vi "Progress Bar Front Panel.vi"(7 "Enable Cancel?":bool, 9 "Main Title":string, 10 "Progress Bar Dialog":refnum<class "Progress Bar Dialog.lvclass">, 11 "Total":i32) -> ()   [LabVIEW 2020, in "Progress Bar Dialog.lvclass"]
uses:
  <vilib>/ProgressBar/Progress Bar Dialog.lvclass
  <vilib>/ProgressBar/Progress Bar Dialog.lvclass/Progress Bar Dialog.ctl
panel:
  in  "Cancelling":string="Cancelling..."
  in  "Progress Format String":string="%d of %s"
  out "Main Heading":string="Working..."
  in  "Cancel":bool
  out "Status Heading":string="0 of 0"
  out "Progress Bar":dbl(slide) scale=0.0..1.0
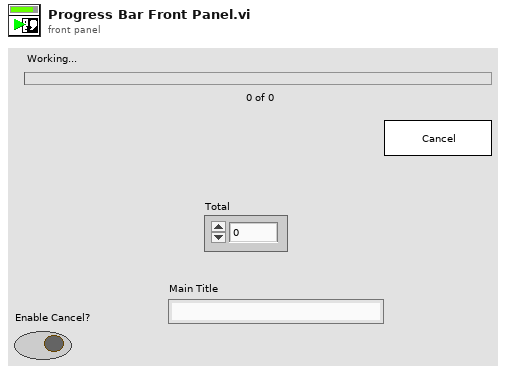
[diagram p1: front panel]
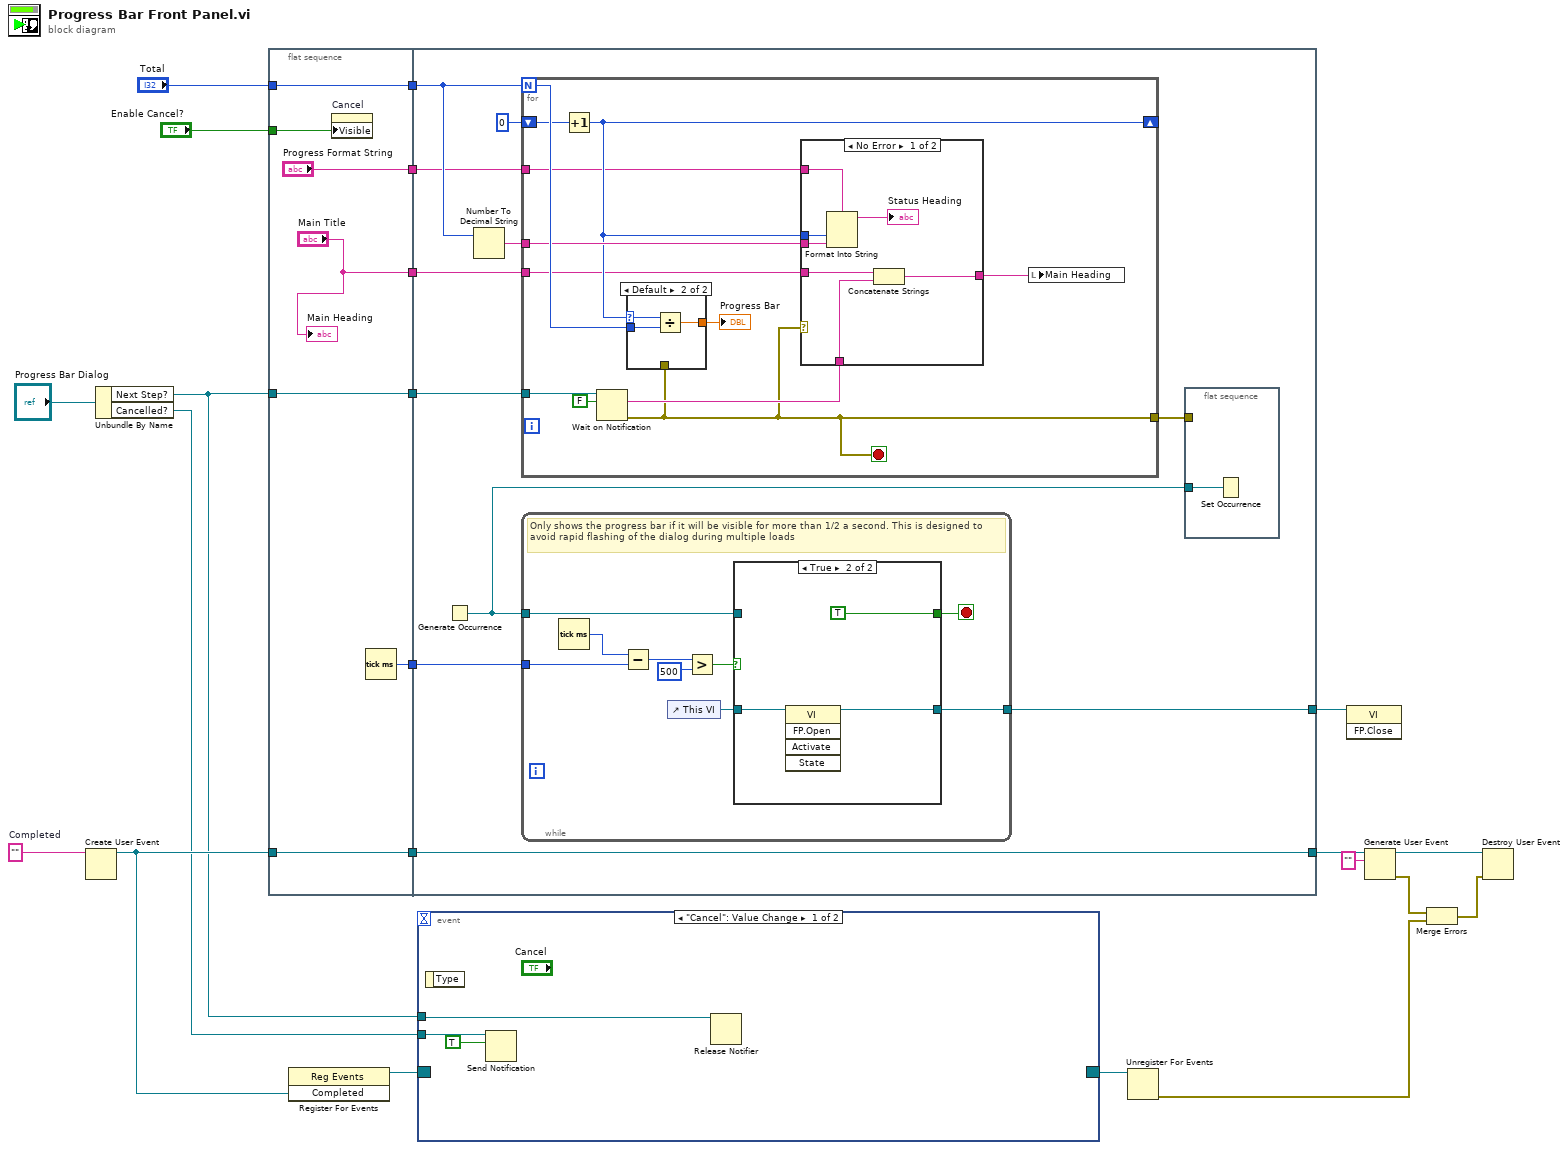
[diagram p0: block diagram]
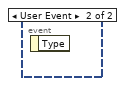
[diagram p2: hidden frame]
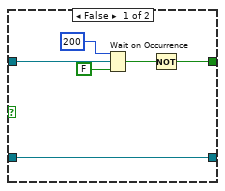
[diagram p3: hidden frame]
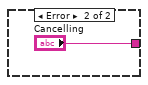
[diagram p4: hidden frame]
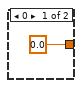
[diagram p5: hidden frame]
diagram:
  w13 = ""  # Completed
  n1 = Create User Event(user event datatype=w13) -> (user event=w15:refnum<user-event>)  [unwired: 1 in, 1 out]
  n2 = Unbundle By Name("Progress Bar Dialog") -> ("Next Step?"=w8:refnum<notifier>, "Cancelled?"=w7:refnum<notifier>)
  n3 = flat-sequence {
    tunnel: [w29] -> w22
    tunnel: [w28] -> w21
    tunnel: "Total" -> [w28]
    tunnel: "Enable Cancel?" -> [w27]
    tunnel: [w26] -> w18
    tunnel: w8 -> [w26]
    tunnel: [w25] -> w16
    tunnel: w15 -> [w25]
    tunnel: ["Progress Format String"] -> w5
    tunnel: ["Main Title"] -> w2
    tunnel: w22 -> [w37]
    tunnel: w21 -> [w36]
    tunnel: w18 -> [w35]
    tunnel: [w34] -> w14
    tunnel: w16 -> [w34]
    tunnel: [w32] -> w6
    tunnel: w5 -> [w31]
    tunnel: w2 -> [w30]
    frame #0 {
      n4 = property on="Cancel" class="Bool"("Visible"=w27) -> ()  [unwired: 2 in, 2 out]
      n5 = Tick Count (ms)() -> (millisecond timer value=w29:u32)
      "Main Heading" <- "Main Title"
    }
    frame #1 {
      n6 = Generate Occurrence() -> (w38:refnum<k4>)
      n7 = Number To Decimal String(number=w36) -> (decimal integer string=w39:string)  [unwired: 1 in]
      n8 = for {
        N: w36 -> [w71]
        shift-right: [w64] -> _
        shift-left: 0 -> [w66]
        tunnel: w35 -> [w69]
        tunnel: w39 -> [w68]
        tunnel: [w60] -> w33
        tunnel: w31 -> [w63]
        tunnel: w30 -> [w62]
        stop <- w60 stop-if-true
        n9 = Increment(x=w66) -> (x+1=w64:i32)
        n10 = Wait on Notification(notifier=w69, ignore previous (F)=FALSE) -> (notification=w65:string, error out=w60:errorcluster)  [unwired: 2 in, 2 out]
        n11 = case shown="Default" w64 {
          selector: w64 -> [_ w83]
          tunnel: w71 -> [_ w82]
          tunnel: [0.0 w81] -> w70
          tunnel: w60 -> [_ _]
          frame 0 {
          }
          frame Default {
            n12 = Divide(x=w83, y=w82) -> (x/y=w81:dbl)
          }
        }
        "Progress Bar" <- w70
        n13 = case shown="No Error" w60 {
          tunnel: w68 -> [w78 _]
          tunnel: w65 -> [w74 _]
          tunnel: w64 -> [w77 _]
          tunnel: w63 -> [w76 _]
          tunnel: w62 -> [w75 _]
          tunnel: [w73 "Cancelling"] -> w61
          frame No Error {
            n14 = Format Into String(format string=w76, w77, w78) -> (resulting string=→"Status Heading":string)  [unwired: 2 in, 1 out]
            n15 = Concatenate Strings(w75, w74) -> (w73:string)
          }
          frame Error {
          }
        }
        n16 = local write "Main Heading"(w61) -> ()
      }
      n17 = while {
        tunnel: w38 -> [w42]
        tunnel: w37 -> [w47]
        tunnel: [w45] -> w32
        stop <- w43 stop-if-true
        # "Only shows the progress bar if it will be visible for more than 1/2 a second. This is designed to avoid rapid flashing of the dialog during multiple loads"
        n18 = Tick Count (ms)() -> (millisecond timer value=w48:u32)
        n19 = Subtract(x=w48, y=w47) -> (x-y=w49:u32)
        n20 = control-ref of="This VI"() -> (w46:refnum<vi>)
        n21 = Greater?(x=w49, y=u32 500) -> (0:w44:bool)
        n22 = case shown="True" w44 {
          tunnel: w46 -> [w56 w59]
          tunnel: [w56 w58] -> w45
          tunnel: [w51 TRUE] -> w43
          tunnel: w42 -> [w53 _]
          frame False {
            n23 = Wait on Occurrence(1:FALSE ("ignore previous (T)"), 2:w53, 3:200 ("ms timeout (-1)")) -> (0:w52:bool)
            n24 = Not(x=w52) -> (.not. x?=w51:bool)
          }
          frame True {
            n25 = invoke class="VI" method="FP.Open"(reference=w59) -> (reference out=w58:refnum<vi>)  [unwired: 4 in, 4 out]
          }
        }
      }
      n26 = flat-sequence {
        tunnel: w38 -> [w41]
        tunnel: w33 -> [_]
        frame #0 {
          n27 = Set Occurrence(w41) -> ()
        }
      }
    }
  }
  n28 = register-events(w15) -> (reference out=w17:refnum<event-registration>)  [unwired: 2 in, 1 out]
  n29 = event shown="[0] \"Cancel\": Value Change" {
    selector: w17 -> [_ _]
    dyn-events: [_ _] -> w4
    timeout: _ -> [_ _]
    tunnel: w8 -> [w86 _]
    tunnel: w7 -> [w84 _]
    event "Cancel": Value Change {
      n30 = event-data() -> ()  [unwired: 1 in, 1 out]
      n31 = Send Notification(notification=TRUE, notifier=w84) -> ()  [unwired: 1 in, 2 out]
      n32 = Release Notifier(notifier=w86) -> ()  [unwired: 2 in, 3 out]
    }
    event User Event {
      n33 = event-data() -> ()  [unwired: 1 in, 1 out]
    }
  }
  n34 = Unregister For Events(event registration refnum=w4) -> (error out=w3:errorcluster)  [unwired: 1 in]
  n35 = invoke class="VI" method="FP.Close"(reference=w6) -> ()  [unwired: 2 in, 3 out]
  n36 = Generate User Event(user event=w14, event data cluster="" ("event data")) -> (user event out=w11:refnum<user-event>, error out=w12:errorcluster)  [unwired: 2 in]
  n37 = Merge Errors(w12, w3) -> (w10:errorcluster)
  n38 = Destroy User Event(user event=w11, error in=w10) -> ()  [unwired: 1 out]
